vi "OPC Server.vi"() -> ()   [LabVIEW 2011]
panel:
  in  "WriteOptimizationDutyCycle":i32
  out "NetworkAdapter":string
  out "EnableDiagnostics":bool
  out "AvailableNetworkAdapters":string
  in  "Stop Button":bool
  out "TotalTagCount":dbl
  out "Time_Second":u32
  out "Time_PM":bool
  out "Time_Minute":u32
  out "Time_Hour24":u32
  out "Time_Hour":u32
  out "ProjectName":string
  out "Time":string
  out "FullProjectName":string
  out "Date_Year4":dbl
  out "Date_Year2":dbl
  out "Date_Month":dbl
  out "Date_Day":dbl
  out "Date":string
  out "ClientCount":dbl
  out "ActiveTagCount":u32
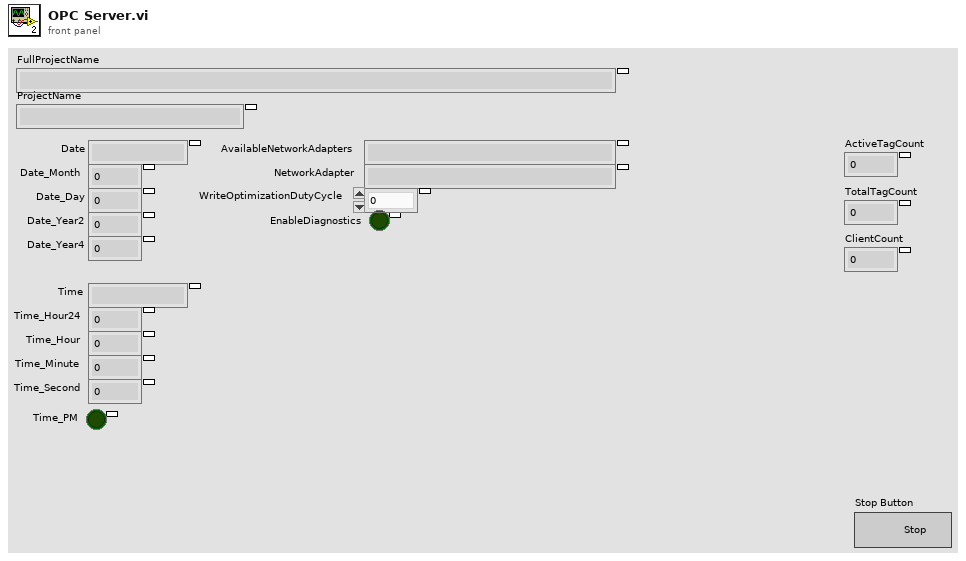
[diagram p1: front panel]
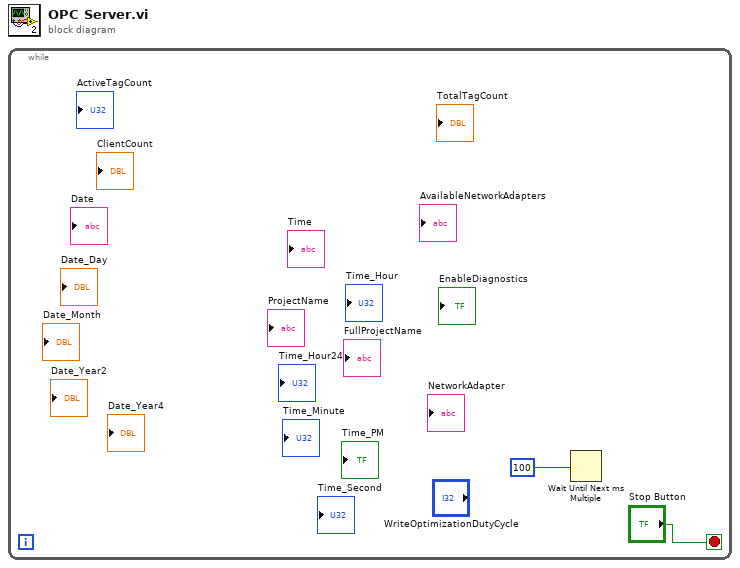
[diagram p0: block diagram]
diagram:
  n1 = while {
    stop <- "Stop Button" stop-if-true
    n2 = Wait Until Next ms Multiple(millisecond multiple=u32 100) -> ()  [unwired: 1 out]
  }
